vi "Channel Count.vi"(8 "error in (no error)":errorcluster, 11 "Plugin Configuration in":refnum<class "Plugin Configuration.lvclass">) -> (0 "error out":errorcluster, 2 "channel count":i32, 3 "Plugin Configuration out":refnum<class "Plugin Configuration.lvclass">)   [LabVIEW 2017, in "DSF Core.lvlib" / "Plugin Configuration.lvclass"]
uses:
  Plugin Configuration.lvclass
  Plugin Configuration.lvclass/Plugin Configuration.ctl
  Thread/Thread Configuration.lvclass
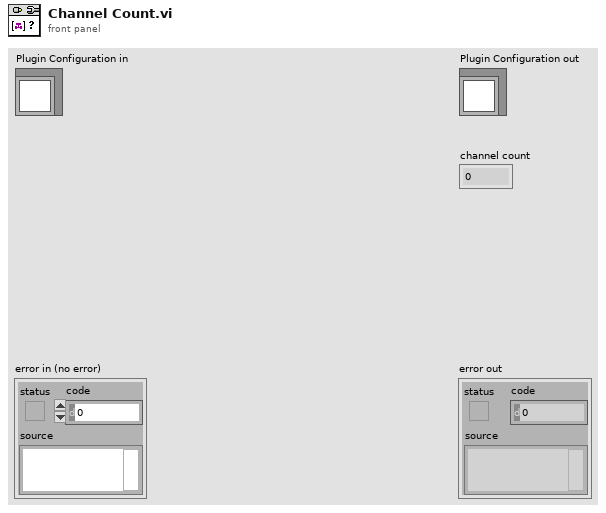
[diagram p1: front panel]
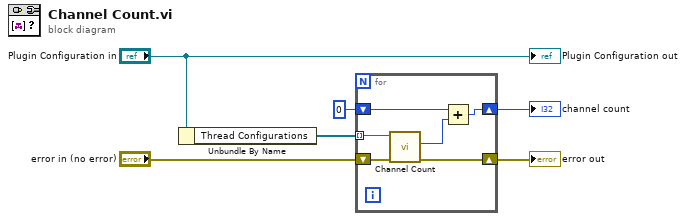
[diagram p0: block diagram]
diagram:
  n1 = Unbundle By Name("Plugin Configuration in") -> ("Thread Configurations"=w5:refnum<class "Thread Configuration.lvclass">[])
  n2 = for {
    shift-right: [w11] -> w2
    shift-left: "error in (no error)" -> [w12]
    tunnel: w5 -> [w10] mode=indexing
    shift-right: [w7] -> w1
    shift-left: 0 ("channel count") -> [w9]
    n3 = call-dynamic "Channel Count.vi"("error in (no error)"=w12, "Thread Configuration in"=w10) -> ("error out"=w11:errorcluster, "channel count"=w8:i32)  [unwired: 7 in, 1 out]
    n4 = Add(x=w9, y=w8) -> (x+y=w7:i32)
  }
  "error out" <- w2
  "channel count" <- w1
  "Plugin Configuration out" <- "Plugin Configuration in"
